vi "Read Binary.vi"(6 "error in (no error)":errorcluster, 8 "timeout ms (1000)":i32=1000, 9 "RawSocket TCP Handler in":refnum<class "RawSocket TCP Handler.lvclass">) -> (0 "error out":errorcluster, 2 "Bytes":u8[](array[numeric]), 3 "RawSocket TCP Handler out":refnum<class "RawSocket TCP Handler.lvclass">)   [LabVIEW 2020, in "wamplv.lvlib" / "RawSocket TCP Handler.lvclass"]
uses:
  RawSocket TCP Handler.lvclass
  C:/local/wamplv/Private/Comm Handlers/TCPSocketBasedCommHandlerBase/TCPSocketBasedCommHandlerBase.lvclass
  TCPSocketBasedCommHandlerBase/TCPSocketBasedCommHandlerBase.lvclass/TCPSocketBasedCommHandlerBase.ctl
  TypeDefs/Message Type.ctl
  TCPSocketBasedCommHandlerBase/Accessors/Read connection ID.vi
  Message Handling/Unpack message frame.vi
  Message Handling/Pack message frame.vi
  <vilib>/Utility/error.llb/Error Cluster From Error Code.vi
  <vilib>/ErrorRing/Error Ring.xnode
  RawSocket TCP Handler.lvclass/RawSocket TCP Handler.ctl
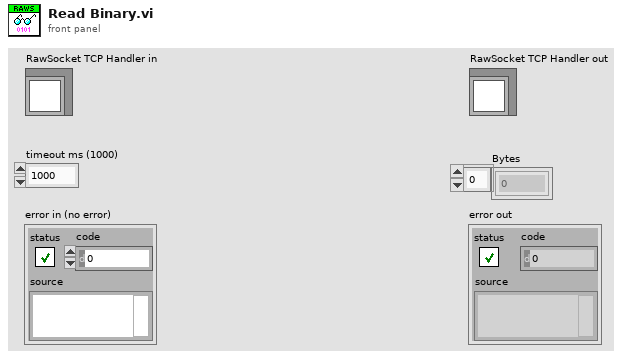
[diagram p1: front panel]
types:
  T1 = typedef "wamplv.lvlib/RawSocket TCP Handler.lvclass/Message Type.ctl" = enum8{"Regular WAMP message", "PING", "PONG"}
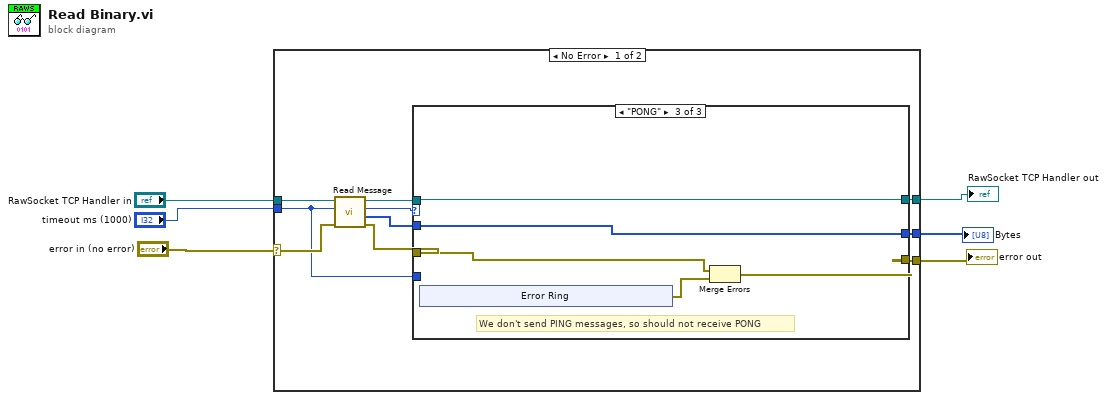
[diagram p0: block diagram]
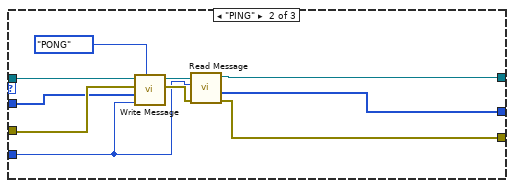
[diagram p3: hidden frame]
diagram:
  n1 = case shown="No Error" "error in (no error)" {
    selector: "error in (no error)" -> [w15 w40]
    tunnel: "RawSocket TCP Handler in" -> [w16 w39]
    tunnel: [w12 _] -> w6
    tunnel: [w10 w40] -> w2
    tunnel: [w9 w39] -> w1
    tunnel: "timeout ms (1000)" -> [w7 _]
    frame No Error {
      n2 = call "Read Message.vi"("error in"=w15, "timeout ms (1000)"=w7, "RawSocket Handler in"=w16) -> ("error out"=w11:errorcluster, "Message data"=w13:u8[], "Message Type"=w14:T1, "RawSocket Handler out"=w8:refnum<class "RawSocket TCP Handler.lvclass">)  [unwired: 3 in]
      n3 = case shown="\"PONG\"" w14 {
        tunnel: [w19 w20 w34] -> w12
        tunnel: w13 -> [w19 w26 w34]
        tunnel: [w17 w22 w30] -> w10
        tunnel: w11 -> [w17 w27 w31]
        tunnel: [w18 w23 w33] -> w9
        tunnel: w8 -> [w18 w29 w33]
        tunnel: w7 -> [_ w21 _]
        frame "Regular WAMP message", Default {
        }
        frame "PING" {
          n4 = call "Write Message.vi"("Message Type"=Message_Type."PONG", "timeout ms (1000)"=w21, "Message"=w26, "error in (no error)"=w27, "RawSocket Handler in"=w29) -> ("error out"=w24:errorcluster, "RawSocket Handler out"=w25:refnum<class "RawSocket TCP Handler.lvclass">)  [unwired: 5 in]
          n5 = call "Read Message.vi"("error in"=w24, "timeout ms (1000)"=w21, "RawSocket Handler in"=w25) -> ("error out"=w22:errorcluster, "Message data"=w20:u8[], "RawSocket Handler out"=w23:refnum<class "RawSocket TCP Handler.lvclass">)  [unwired: 3 in, 1 out]
        }
        frame "PONG" {
          # "We don't send PING messages, so should not receive PONG"
          n6 = xnode "Error Ring"() -> ("error out"=w32:errorcluster)
          n7 = Merge Errors(w31, w32) -> (w30:errorcluster)
        }
      }
    }
    frame Error {
    }
  }
  "error out" <- w2
  "RawSocket TCP Handler out" <- w1
  "Bytes" <- w6
